vi "Meandr_4110.vi"() -> ()   [LabVIEW 2018]
uses:
  <instrlib>/niDCPower/nidcpower.llb/niDCPower Source Mode.ctl
  <instrlib>/niDCPower/nidcpower.llb/niDCPower Wait For Event - Event.ctl
  <instrlib>/niDCPower/nidcpower.llb/niDCPower Output Function.ctl
panel:
  out "Path 2":path
  in  "Path":path
  in  "Коэффициент заполнения,%":dbl
  in  "Source Delay (Sec) 4":dbl=0.1 caption="Source Delay (Sec)" format="%.3p"
  out "Waveform Current 2":dbl[](graph)
  out "Waveform Voltage  2":dbl[](graph)
  out "Voltage Measurement 4":dbl caption="Voltage Measurement"
  out "Current Measurement 4":dbl caption="Current Measurement"
  out "Compliance/Limit Reached 4":bool caption="Compliance/Limit Reached"
  in  "Current Limit Range 4":dbl=0.01 caption="Current Limit Range" format="%.3p"
  in  "Voltage Level Range 4":dbl=6.0 caption="Voltage Level Range" format="%.5p"
  in  "Current Limit 4":dbl=0.01 caption="Current Limit" format="%.3p"
  in  "Channel Name 4":string="0" caption="Channel Name"
  in  "Resource Name 4":refnum<k15>="Dev1" caption="Resource Name"
  out "Актуальное время":string
  in  "Voltage level":dbl
  out "Numeric 3":i32
  out "Время без импульса, сек":dbl
  out "Время импульса, сек":dbl
  out "Скважность":dbl
  in  "Период импульса, сек":dbl
  out "Waveform Chart":dbl(graph)
  out "Множитель":dbl
  in  "Остановка цикла":bool
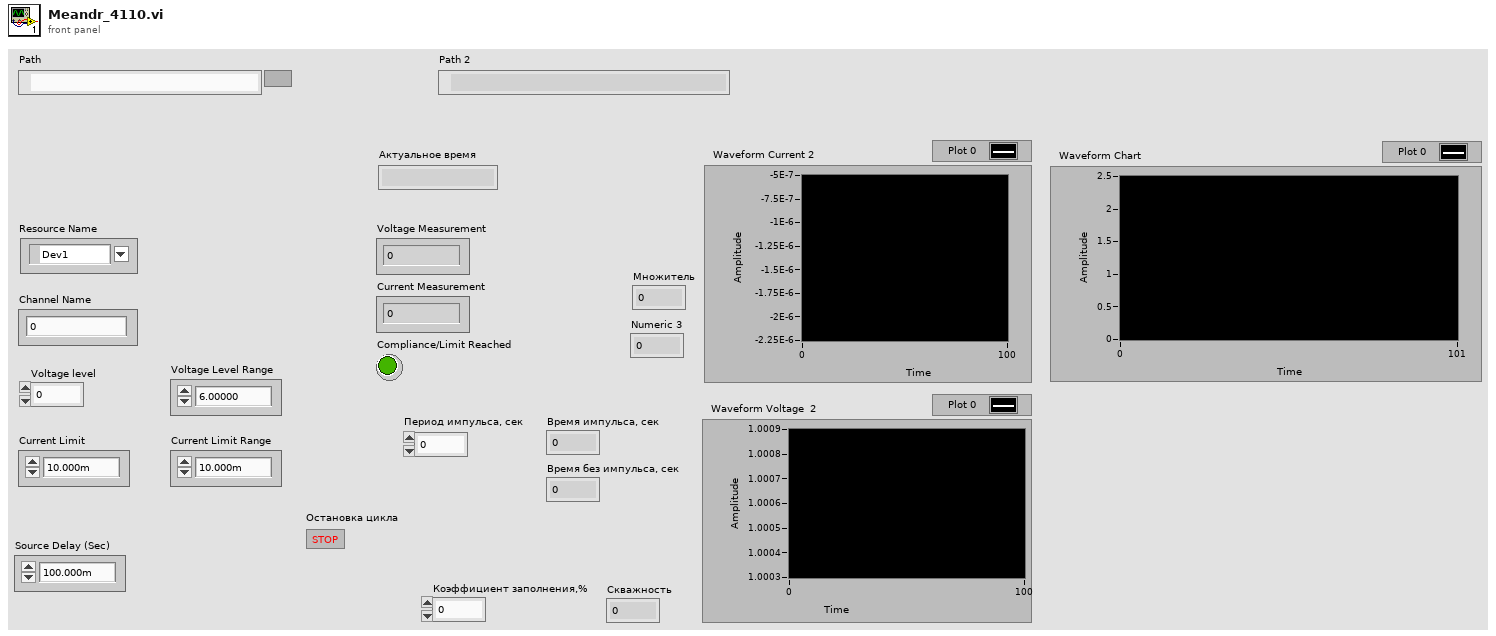
[diagram p1: front panel]
types:
  T1 = enum16{"open", "replace", "create", "open or create", "replace or create", "replace or create with confirmation"}
  T2 = typedef "niDCPower Output Function.ctl" = i32
  T3 = typedef "niDCPower Wait For Event - Event.ctl" = i32
  T4 = typedef "niDCPower Source Mode.ctl" = i32
  T5 = typedef "LVDateTimeRec.ctl" = cluster{"fractional second":dbl, "second":i32, "minute":i32, "hour":i32, "day of month":i32, "month":i32, "year":i32, "day of week":i32, "day of year":i32, "DST":i32}
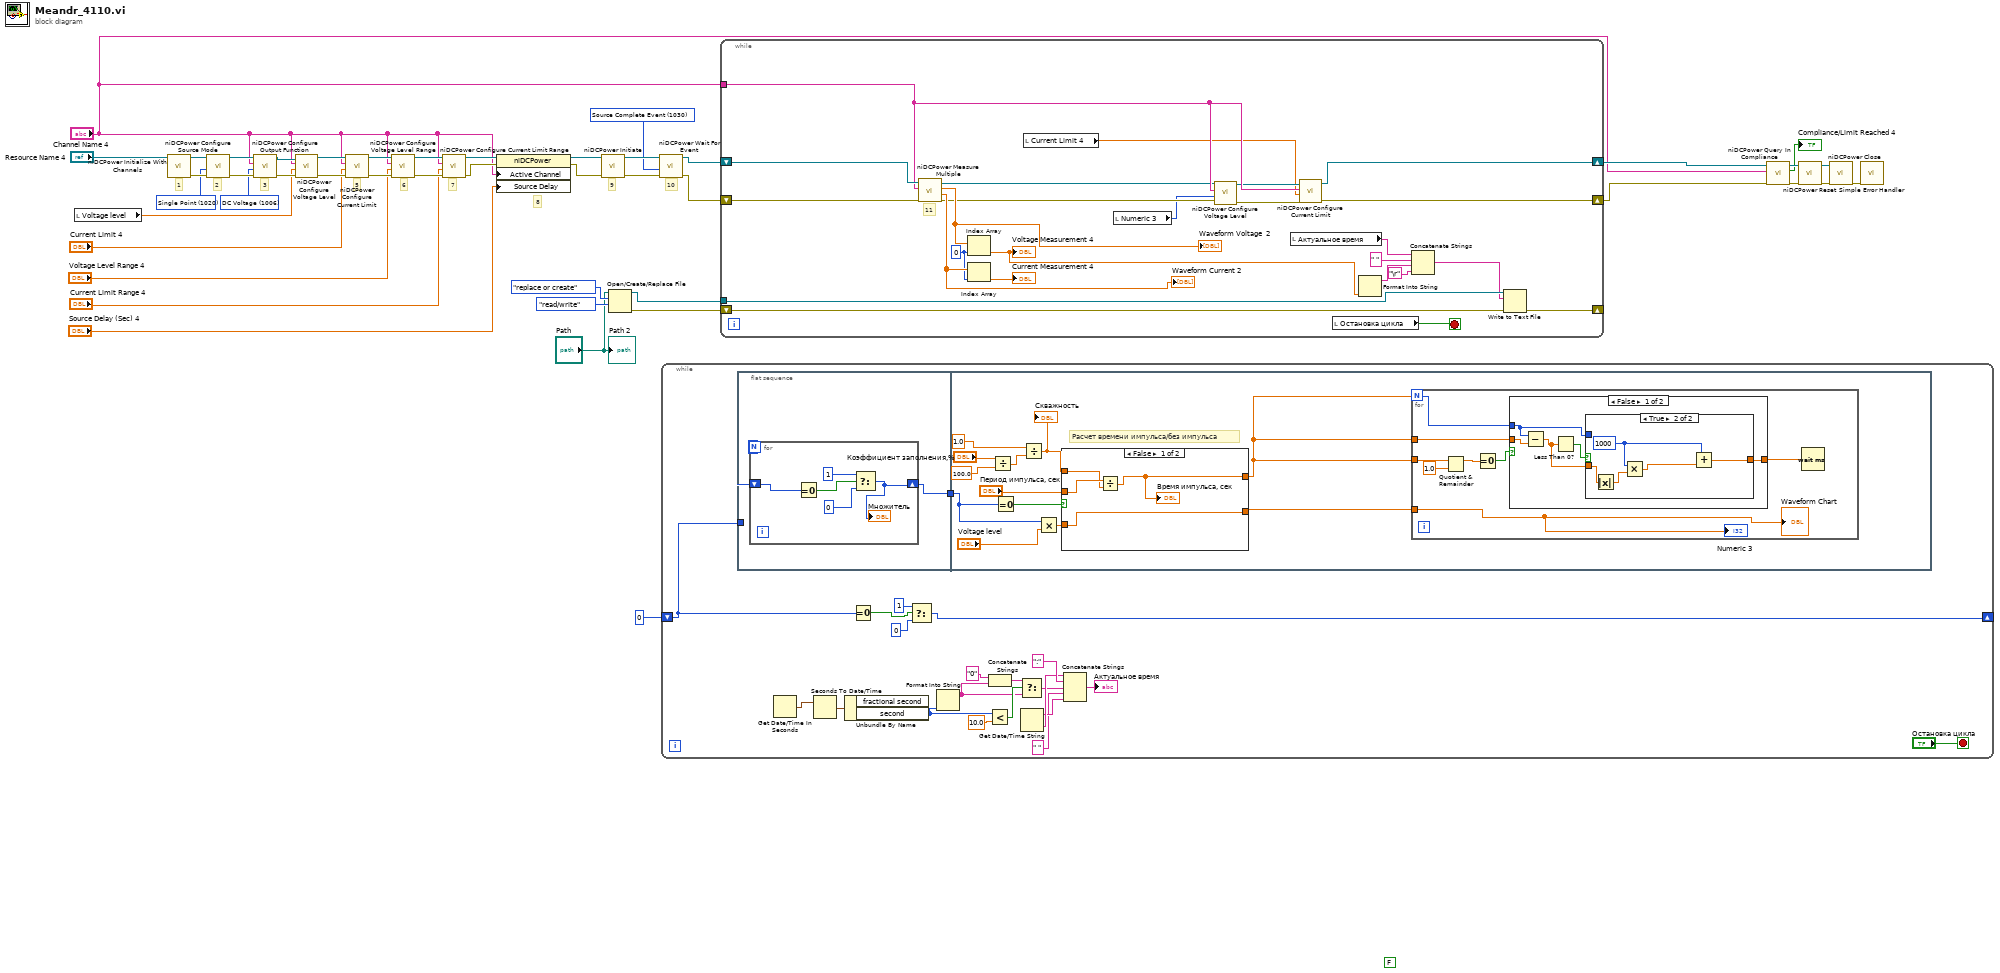
[diagram p0: block diagram]
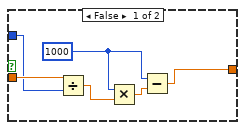
[diagram p2: hidden frame]
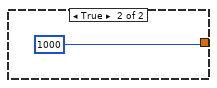
[diagram p3: hidden frame]
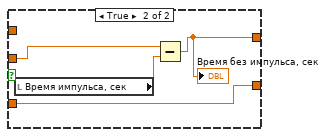
[diagram p4: hidden frame]
diagram:
  w20 = T2 1006 items=["DC Voltage"=1006, "DC Current"=1007, "Pulse Voltage"=1049, "Pulse Current"=1050] ("output function")
  w23 = T3 1030 items=["Source Complete Event"=1030, "Measure Complete Event"=1031, "Sequence Iteration Complete Event"=1032, "Sequence Engine Done Event"=1033] ("event")
  w35 = T4 1020 items=["Single Point"=1020, "Sequence"=1021] ("source mode")
  (unwired) FALSE
  # "9"
  # "10"
  # "7"
  # "6"
  # "2"
  # "3"
  # "8"
  # "5"
  # "1"
  n1 = local read "Voltage level"() -> (w6:dbl)
  n2 = call <instrlib>:"niDCPower Initialize With Channels.vi"("resource name"="Resource Name 4") -> ("error out"=w39:errorcluster, "instrument handle out"=w38:refnum<k15>)  [unwired: 3 in, 6 out]
  n3 = call <instrlib>:"niDCPower Configure Source Mode.vi"("error in (no error)"=w39, "source mode"=w35, "instrument handle"=w38) -> ("error out"=w37:errorcluster, "instrument handle out"=w36:refnum<k15>)  [unwired: 7 out]
  n4 = call <instrlib>:"niDCPower Configure Output Function.vi"("error in (no error)"=w37, "output function"=w20, "channel name"="Channel Name 4", "instrument handle"=w36) -> ("error out"=w21:errorcluster, "instrument handle out"=w22:refnum<k15>)  [unwired: 6 out]
  n5 = call <instrlib>:"niDCPower Configure Voltage Level.vi"("error in (no error)"=w21, "voltage level"=w6, "channel name"="Channel Name 4", "instrument handle"=w22) -> ("error out"=w41:errorcluster, "instrument handle out"=w42:refnum<k15>)  [unwired: 6 out]
  n6 = call <instrlib>:"niDCPower Configure Current Limit.vi"("error in (no error)"=w41, "current limit"="Current Limit 4", "channel name"="Channel Name 4", "instrument handle"=w42) -> ("error out"=w34:errorcluster, "instrument handle out"=w33:refnum<k15>)  [unwired: 1 in, 5 out]
  n7 = call <instrlib>:"niDCPower Configure Voltage Level Range.vi"("error in (no error)"=w34, "voltage level range"="Voltage Level Range 4", "channel name"="Channel Name 4", "instrument handle"=w33) -> ("error out"=w32:errorcluster, "instrument handle out"=w31:refnum<k15>)  [unwired: 6 out]
  n8 = call <instrlib>:"niDCPower Configure Current Limit Range.vi"("error in (no error)"=w32, "current limit range"="Current Limit Range 4", "channel name"="Channel Name 4", "instrument handle"=w31) -> ("error out"=w26:errorcluster, "instrument handle out"=w29:refnum<k15>)  [unwired: 6 out]
  n9 = property class="niDCPower"(reference=w29, error in=w26, "Active Channel"="Channel Name 4", "Source Delay"="Source Delay (Sec) 4") -> (reference out=w28:refnum<k15>, error out=w27:errorcluster)
  n10 = call <instrlib>:"niDCPower Initiate.vi"("error in (no error)"=w27, "instrument handle"=w28) -> ("error out"=w24:errorcluster, "instrument handle out"=w25:refnum<k15>)  [unwired: 2 in, 6 out]
  n11 = Open/Create/Replace File(file path (use dialog)="Path", operation (0:open)=T1."replace or create", access (0:read/write)=enum16{"read/write", "read-only", "write-only"}."read/write") -> (refnum out=w2:refnum<file>, error out=w1:errorcluster)  [unwired: 3 in, 1 out]
  n12 = call <instrlib>:"niDCPower Wait For Event.vi"("error in (no error)"=w24, "event"=w23, "instrument handle"=w25) -> ("error out"=w11:errorcluster, "instrument handle out"=w10:refnum<k15>)  [unwired: 1 in, 6 out]
  n13 = while {
    shift-right: [w59] -> _
    shift-left: 0 -> [w61]
    stop <- "Остановка цикла" stop-if-true
    n14 = flat-sequence {
      tunnel: [w66] -> w65
      tunnel: w61 -> [w67]
      tunnel: w65 -> [w82]
      frame #0 {
        n15 = for {
          N: 1 -> [_]
          shift-right: [w69] -> w66
          shift-left: w67 -> [w70]
          n16 = Equal To 0?(x=w70) -> (x = 0?=w72:bool)
          n17 = Select(t=1, s=w72, f=0) -> (s? t:f=w69:i32)
          "Множитель" <- w69
        }
      }
      frame #1 {
        # "Расчет времени импульса/без импульса"
        n18 = Divide(x="Коэффициент заполнения,%", y=100.0) -> (x/y=w78:dbl)
        n19 = Equal To 0?(x=w82) -> (x = 0?=w85:bool)
        n20 = Divide(x=1.0, y=w78) -> (x/y=w75:dbl)
        "Скважность" <- w75
        n21 = Multiply(x=w82, y="Voltage level") -> (x*y=w84:dbl)
        n22 = case shown="False" w85 {
          tunnel: [w113 w117] -> w74
          tunnel: [w114 w118] -> w83
          tunnel: w84 -> [w114 w118]
          tunnel: "Период импульса, сек" -> [w112 w115]
          tunnel: w75 -> [w111 _]
          frame False {
            n23 = Divide(x=w112, y=w111) -> (x/y=w113:dbl)
            "Время импульса, сек" <- w113
          }
          frame True {
            n24 = local read "Время импульса, сек"() -> (w116:dbl)
            n25 = Subtract(x=w115, y=w116) -> (x-y=w117:dbl)
            "Время без импульса, сек" <- w117
          }
        }
        n26 = for {
          N: w74 -> [w88]
          tunnel: w83 -> [w93]
          tunnel: w74 -> [w87]
          tunnel: w74 -> [w89]
          n27 = Quotient & Remainder(x=w87, y=1.0) -> (x-y*floor(x/y)=w91:dbl)  [unwired: 1 out]
          n28 = Equal To 0?(x=w91) -> (x = 0?=w90:bool)
          n29 = case shown="False" w90 {
            tunnel: [w95 u32 1000 ("milliseconds to wait")] -> w92
            tunnel: w89 -> [w98 _]
            tunnel: w88 -> [w94 _]
            frame False {
              n30 = Subtract(x=w94, y=w98) -> (x-y=w96:dbl)
              n31 = Less Than 0?(x=w96) -> (x < 0?=w97:bool)
              n32 = case shown="True" w97 {
                tunnel: w96 -> [w104 w109]
                tunnel: [w102 w108] -> w95
                tunnel: w94 -> [w103 _]
                frame False {
                  w100 = 1000
                  n33 = Divide(x=w104, y=w103) -> (x/y=w99:dbl)
                  n34 = Multiply(x=w100, y=w99) -> (x*y=w101:dbl)
                  n35 = Subtract(x=w100, y=w101) -> (x-y=w102:dbl)
                }
                frame True {
                  w105 = 1000
                  n36 = Absolute Value(x=w109) -> (abs(x)=w106:dbl)
                  n37 = Multiply(x=w105, y=w106) -> (x*y=w107:dbl)
                  n38 = Add(x=w105, y=w107) -> (x+y=w108:dbl)
                }
              }
            }
            frame True {
            }
          }
          n39 = Wait (ms)(milliseconds to wait=w92) -> ()  [unwired: 1 out]
          "Waveform Chart" <- w93
          "Numeric 3" <- w93
        }
      }
    }
    n40 = Get Date/Time In Seconds() -> (seconds since 1Jan1904=w54:timestamp)
    n41 = Seconds To Date/Time(time stamp (now)=w54) -> (date time rec=w55:T5)  [unwired: 1 in]
    n42 = Unbundle By Name(w55) -> ("second"=w48:i32)  [unwired: 1 out]
    n43 = Equal To 0?(x=w61) -> (x = 0?=w63:bool)
    n44 = Select(t=1, s=w63, f=0) -> (s? t:f=w59:i32)
    n45 = Format Into String(w48) -> (resulting string=w46:string)  [unwired: 3 in, 1 out]
    n46 = Concatenate Strings("0", w46) -> (w45:string)
    n47 = Less?(x=w48, y=10.0) -> (x < y?=w50:bool)
    n48 = Select(t=w45, s=w50, f=w46) -> (s? t:f=w49:string)
    n49 = Get Date/Time String() -> (date string=w53:string, time string=w56:string)  [unwired: 3 in]
    n50 = Concatenate Strings(w56, ":" ("string"), w49, " " ("string"), w53) -> (→"Актуальное время":string)
  }
  n51 = while {
    tunnel: "Channel Name 4" -> [w140]
    shift-right: [w141] -> w9
    shift-left: w11 -> [w143]
    shift-right: [w139] -> w8
    shift-left: w10 -> [w142]
    tunnel: w2 -> [w127]
    shift-right: [w119] -> _
    shift-left: w1 -> [w120]
    stop <- w130 stop-if-true
    w135 = 0 ("index")
    # "11"
    n52 = call <instrlib>:"niDCPower Measure Multiple.vi"("error in (no error)"=w143, "channel name"=w140, "instrument handle"=w142) -> ("error out"=w134:errorcluster, "current measurements"=w137:dbl[], "voltage measurements"=w138:dbl[], "instrument handle out"=w132:refnum<k15>)  [unwired: 5 out]
    "Waveform Voltage  2" <- w138
    "Waveform Current 2" <- w137
    n53 = Index Array "Index Array"(array=w138, index=w135) -> (element=w125:dbl)
    "Voltage Measurement 4" <- w125
    n54 = Index Array(array=w137, index=w135) -> (element=→"Current Measurement 4":dbl)
    n55 = local read "Current Limit 4"() -> (w128:dbl)
    n56 = local read "Numeric 3"() -> (w129:i32)
    n57 = call <instrlib>:"niDCPower Configure Voltage Level.vi"("error in (no error)"=w134, "voltage level"=w129, "channel name"=w140, "instrument handle"=w132) -> ("error out"=w133:errorcluster, "instrument handle out"=w131:refnum<k15>)  [unwired: 6 out]
    n58 = local read "Актуальное время"() -> (w126:string)
    n59 = call <instrlib>:"niDCPower Configure Current Limit.vi"("error in (no error)"=w133, "current limit"=w128, "channel name"=w140, "instrument handle"=w131) -> ("error out"=w141:errorcluster, "instrument handle out"=w139:refnum<k15>)  [unwired: 1 in, 5 out]
    n60 = local read "Остановка цикла"() -> (w130:bool)
    n61 = Format Into String(w125) -> (resulting string=w123:string)  [unwired: 3 in, 1 out]
    n62 = Concatenate Strings(w126, " " ("string"), w123, "\r") -> (w124:string)
    n63 = Write to Text File(file (use dialog)=w127, text=w124, error in=w120) -> (error out=w119:errorcluster)  [unwired: 1 in, 2 out]
  }
  n64 = call <instrlib>:"niDCPower Query In Compliance.vi"("error in (no error)"=w9, "channel name"="Channel Name 4", "instrument handle"=w8) -> ("error out"=w14:errorcluster, "in compliance?"=→"Compliance/Limit Reached 4":bool, "instrument handle out"=w17:refnum<k15>)  [unwired: 6 out]
  n65 = call <instrlib>:"niDCPower Reset.vi"("error in (no error)"=w14, "instrument handle"=w17) -> ("error out"=w15:errorcluster, "instrument handle out"=w16:refnum<k15>)  [unwired: 2 in, 6 out]
  n66 = call <instrlib>:"niDCPower Close.vi"("error in (no error)"=w15, "instrument handle"=w16) -> ("error out"=w13:errorcluster)  [unwired: 9 out]
  n67 = call <vilib>:"Simple Error Handler.vi"("error in (no error)"=w13) -> ()  [unwired: 1 in, 8 out]
  "Path 2" <- "Path"
